vi "4.2.vi"() -> ()   [LabVIEW 2013]
panel:
  out "Numeric 2":dbl
  in  "Numeric":i32
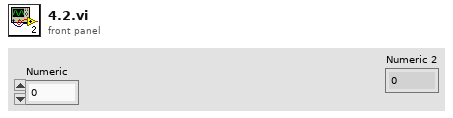
[diagram p1: front panel]
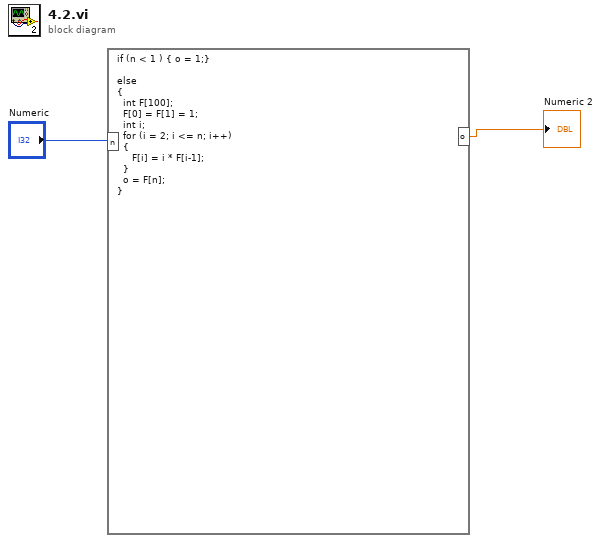
[diagram p0: block diagram]
diagram:
  n1 = formula code="if (n < 1 ) { o = 1;}\n\nelse \n{\n  int F[100];\n  F[0] = F[1] = 1;\n  int i;\n  for (i = 2; i <= n; i++)\n  {\n     F[i] = i * F[i-1];\n  }\n  o = F[n];\n}"("n"="Numeric") -> ("o"=→"Numeric 2":dbl)
